vi "oa_Extract Even Angle Signal by Indice.vi"   [LabVIEW 2017, in "SoundVib_OAUtility.lvlib"]
uses:
  <vilib>/addons/Sound and Vibration/Order Analysis/Utility/SoundVib_OAUtility.lvlib
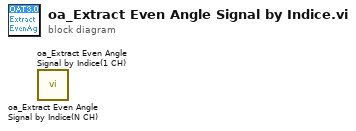
[diagram p0: block diagram]
diagram:
  n1 = call <vilib>:"oa_Extract Even Angle Signal by Indice(N CH).vi"() -> ()  [unwired: 12 in, 4 out]
  n2 = call <vilib>:"oa_Extract Even Angle Signal by Indice(1 CH).vi"() -> ()  [unwired: 12 in, 4 out]
